vi "Drive Teleop Handler.vi"(10 "Call Context":T1) -> ()   [LabVIEW 2025]
uses:
  swerve-template/Type Definitions/Data/Robot Velocities.ctl
  <vilib>/Rock Robotics/WPI/DriverStation/WPI_DriverStationDerivedRobotMode.ctl
  Drive/Implementation/Driving Mode.ctl
  <vilib>/Rock Robotics/WPI/Joystick/XBox Buttons Indexer.ctl
  ce51abe2-3967-49ec-91df-d4b8ef358bb3.vi
  20f039dc-a6f5-4e97-88ba-31848a91c715.vi
  fdc21bd4-9215-41b8-8367-bf19dde4ba27.vi
  2558f998-dd4e-4154-8f44-6f70b21d0474.vi
  <vilib>/Rock Robotics/WPI/Utilities/WPI_GetSetVariantRefNum.vi
  <vilib>/Rock Robotics/Network Tables/NT Read Number.vi
  <vilib>/Rock Robotics/Network Tables/NT Read Boolean.vi
  Framework/Robot Global Data.vi
  <vilib>/Rock Robotics/Network Tables/NT Write Boolean.vi
panel:
  in  "Max Translation Align":dbl=4.0
  in  "Deadband Info":T2={"Deadband"=0.05, "Deadband High"=1.0, "Deadband Low"=0.05}
  in  "Max Velocities":T3={"X Velocity"=15.0, "Y Velocity"=15.0, "Rotational \nVelocity"=270.0}
  in  "Sinusoidal Terms":cluster{"Max Velocity":dbl, "Frequency":dbl}
  in  "Teleop Mode":T4(ring)
  in  "Joystick Inputs":T5(array[cluster])
  in  "Send Inputs":bool
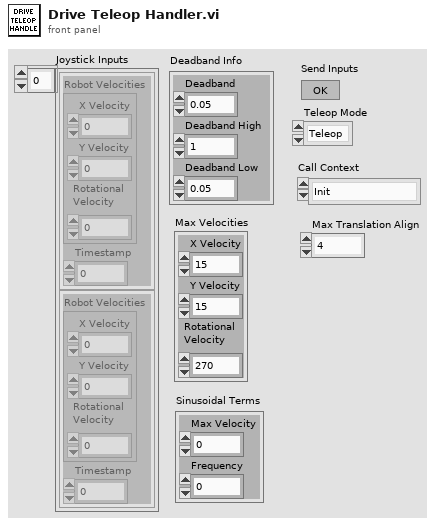
[diagram p1: front panel]
types:
  T1 = typedef "WPI_DriverStationDerivedRobotMode.ctl" = enum16{"Init", "Execute", "Stop"}
  T2 = cluster{"Deadband":dbl, "Deadband High":dbl, "Deadband Low":dbl}
  T3 = typedef "Robot Velocities.ctl" = cluster{"X Velocity":dbl, "Y Velocity":dbl, "Rotational \nVelocity":dbl}
  T4 = enum16{"Teleop", "Simulated Teleop", "Sine Velocity Profiles", "Circle Simulator"}
  T5 = cluster{"Robot Velocities":T3, "Timestamp":dbl}[]
  T6 = typedef "XBox Buttons Indexer.ctl" = enum16{"A", "B", "X", "Y", "Left Bumper", "Right Bumper", "Back", "Start", "Left Joystick", "Right Joystick"}
  T7 = typedef "Driving Mode.ctl" = enum16{"Robot Centric", "Field Centric"}
  T8 = typedef "WPI_JoystickDevRef.ctl" = cluster{"Device":T9}
  T9 = typedef "WPI_JoystickDeviceEnum.ctl" = enum16{"USB 0", "USB 1", "USB 2", "USB 3", "USB 4", "USB 5"}
  T10 = typedef "CTRE_PigeonIMU_DeviceRef.ctl" = cluster{"DeviceStatus":errorcluster, "Device Number":u8, "Type":T11, "Device ID":u32, "Handle":u64, "UsageFrame":u32, "Library Path":path}
  T11 = typedef "CTRE_PigeonIMU_ConnectionType.ctl" = u32
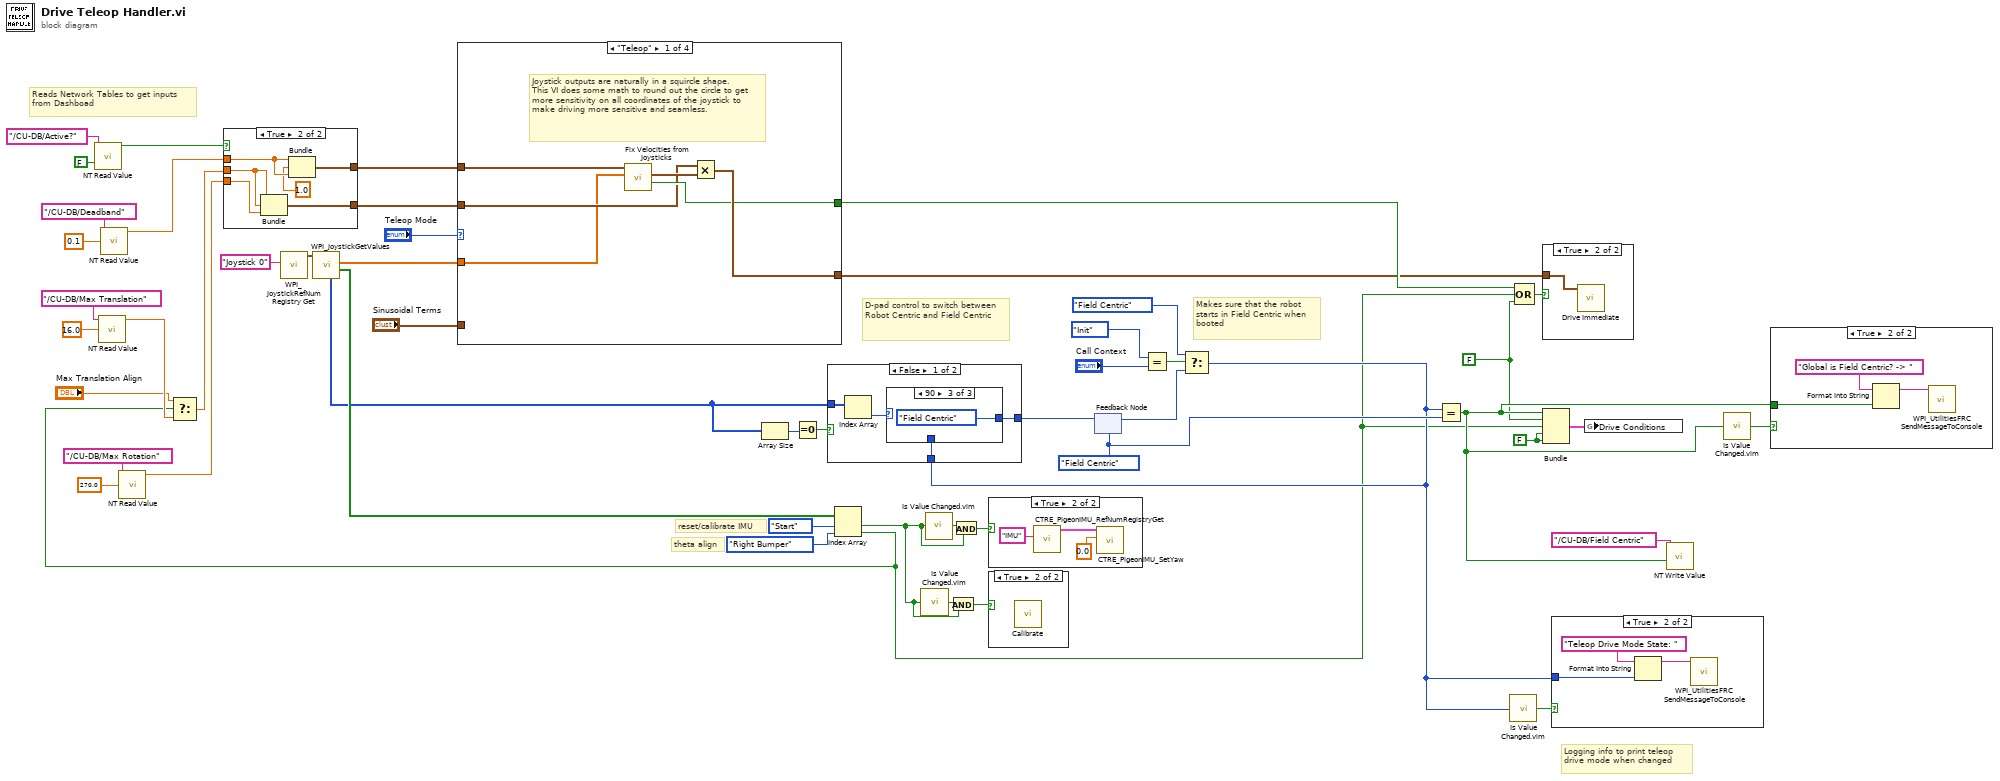
[diagram p0: block diagram]
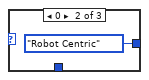
[diagram p7: hidden frame]
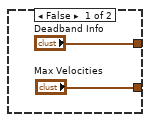
[diagram p9: hidden frame]
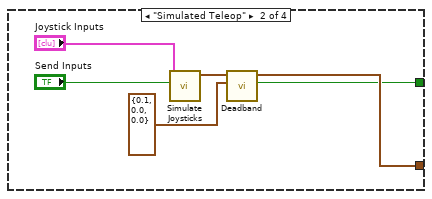
[diagram p10: hidden frame]
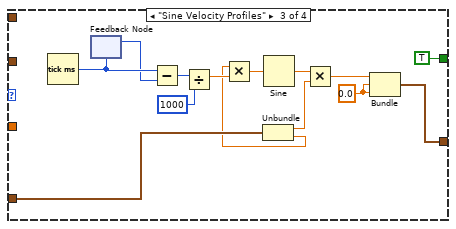
[diagram p11: hidden frame]
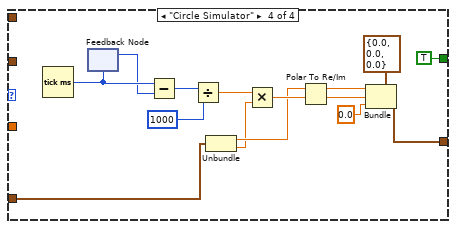
[diagram p12: hidden frame]
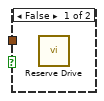
[diagram p13: hidden frame]
diagram:
  w6 = FALSE
  w5 = FALSE
  w18 = Driving_Mode."Field Centric"
  # "theta align"
  # "reset/calibrate IMU"
  # "Reads Network Tables to get inputs from Dashboad"
  # "Logging info to print teleop drive mode when changed"
  # "Makes sure that the robot starts in Field Centric when booted"
  # "D-pad control to switch between Robot Centric and Field Centric"
  n1 = call-poly <vilib>:"NT Read Value.vi"("default value"=FALSE ("Default Value"), "name"="/CU-DB/Active?" ("Name")) -> ("value"=w33:bool)  [unwired: 7 in, 2 out]
  n2 = call-poly <vilib>:"NT Read Value.vi"("default value"=16.0 ("Default Value"), "name"="/CU-DB/Max Translation" ("Name")) -> ("value"=w3:dbl)  [unwired: 7 in, 2 out]
  n3 = call-poly <vilib>:"NT Read Value.vi"("default value"=0.1 ("Default Value"), "name"="/CU-DB/Deadband" ("Name")) -> ("value"=w32:dbl)  [unwired: 7 in, 2 out]
  n4 = call-poly <vilib>:"NT Read Value.vi"("default value"=270.0 ("Default Value"), "name"="/CU-DB/Max Rotation" ("Name")) -> ("value"=w30:dbl)  [unwired: 7 in, 2 out]
  n5 = call <vilib>:"WPI_JoystickRefNum Registry Get.vi"("refnum name"="Joystick 0") -> ("JoystickDevRef"=w50:T8)  [unwired: 1 in, 9 out]
  n6 = call <vilib>:"WPI_JoystickGetValues.vi"("JoystickDevRef"=w50) -> ("Buttons"=w47:bool[], "Axes"=w49:dbl[], "POVs"=w25:i16[])  [unwired: 6 in, 2 out]
  n7 = Array Size(array=w25) -> (size(s)=w24:i32)
  n8 = Equal To 0?(x=w24) -> (x = 0?=w23:bool)
  n9 = Index Array(array=w47, index #1=XBox_Buttons_Indexer."Start" ("XBox Buttons"), index #2=XBox_Buttons_Indexer."Right Bumper" ("XBox Buttons")) -> (element #1=w10:bool, element #2=w2:bool)
  n10 = Select(t="Max Translation Align", s=w2, f=w3) -> (s? t:f=w4:dbl)
  n11 = case shown="True" w33 {
    tunnel: w32 -> [_ w59]
    tunnel: ["Deadband Info" w57] -> w31
    tunnel: w4 -> [_ w56]
    tunnel: w30 -> [_ w55]
    tunnel: ["Max Velocities" w54] -> w29
    frame False {
    }
    frame True {
      n12 = Bundle("value"=w56, "value"=w56, "value"=w55) -> (w54:cluster{"value":dbl, "value":dbl, "value":dbl})  [unwired: 1 in]
      n13 = Bundle("value"=w59, "value"=1.0, "value"=w59) -> (w57:cluster{"value":dbl, "value":dbl, "value":dbl})  [unwired: 1 in]
    }
  }
  n14 = case shown="\"Teleop\"" "Teleop Mode" {
    tunnel: w49 -> [w60 _ _ _]
    tunnel: [w65 w71 w76 w98] -> w8
    tunnel: "Sinusoidal Terms" -> [_ _ w75 w88]
    tunnel: w31 -> [w64 _ _ _]
    tunnel: w29 -> [w61 _ _ _]
    tunnel: [w62 w66 TRUE ("Sending Input?") TRUE ("Sending Input?")] -> w27
    frame "Teleop" {
      # "Joystick outputs are naturally in a squircle shape.\nThis VI does some math to round out the circle to get more sensitivity on all coordinates of the joystick to make driving more sensitive and seamless."
      n15 = call "Fix Velocities from Joysticks.vi"("Axes"=w60, "Deadband"=w64) -> ("Sending Input?"=w62:bool, "Adjusted Robot Velocities"=w63:T3)  [unwired: 8 in]
      n16 = Multiply(x=w61, y=w63) -> (x*y=w65:T3)
    }
    frame "Simulated Teleop" {
      n17 = call "Simulate Joysticks.vi"("Send Inputs"="Send Inputs", "Joystick Inputs"="Joystick Inputs") -> ("Joystick Inputs"=w68:T3)  [unwired: 9 in]
      n18 = call "Deadband.vi"("Deadband Info"=T2 {"Deadband"=0.1, "Deadband High"=0.0, "Deadband Low"=0.0}, "Robot Velocities"=w68) -> ("Sending Input?"=w66:bool, "Adjusted Robot Velocities"=w71:T3)  [unwired: 8 in]
    }
    frame "Sine Velocity Profiles" {
      w84 = 0.0
      n19 = Tick Count (ms)() -> (millisecond timer value=w78:u32)
      n20 = feedback #1(w78) -> (w77:u32)
      n21 = feedback-in #1(w77) -> ()
      n22 = Subtract(x=w78, y=w77) -> (x-y=w82:u32)
      n23 = Divide(x=w82, y=u32 1000) -> (x/y=w80:dbl)
      n24 = Unbundle(w75) -> ("Max Velocity"=w73:dbl, "Frequency"=w74:dbl)
      n25 = Multiply(x=w74, y=w80) -> (x*y=w79:dbl)
      n26 = Sine(x=w79) -> (sin(x)=w83:dbl)
      n27 = Multiply(x=w83, y=w73) -> (x*y=w85:dbl)
      n28 = Bundle(w85, w84, w84) -> (w76:cluster{dbl, dbl, dbl})  [unwired: 1 in]
    }
    frame "Circle Simulator" {
      n29 = Tick Count (ms)() -> (millisecond timer value=w94:u32)
      n30 = feedback #2(w94) -> (w93:u32)
      n31 = feedback-in #2(w93) -> ()
      n32 = Subtract(x=w94, y=w93) -> (x-y=w96:u32)
      n33 = Divide(x=w96, y=u32 1000) -> (x/y=w90:dbl)
      n34 = Unbundle(w88) -> ("Max Velocity"=w91:dbl, "Frequency"=w89:dbl)
      n35 = Multiply(x=w90, y=w89) -> (x*y=w92:dbl)
      n36 = Polar To Re/Im(2:w92, 3:w91) -> (0:w86:dbl, 1:w87:dbl)
      n37 = Bundle(cluster=T3 {"X Velocity"=0.0, "Y Velocity"=0.0, "Rotational \nVelocity"=0.0} ("Robot Velocities (ft/s and deg/s)"), "X Velocity"=w87, "Y Velocity"=w86, "Rotational \nVelocity"=0.0 ("Rotational \nVelocity")) -> (w98:T3)
    }
  }
  n38 = call "Is Value Changed.vim"("value"=w10) -> ("changed or first call?"=w13:bool)
  n39 = call "Is Value Changed.vim"("value"=w10) -> ("changed or first call?"=w45:bool)
  n40 = And(x=w13, y=w10) -> (x .and. y?=w12:bool)
  n41 = And(x=w45, y=w10) -> (x .and. y?=w44:bool)
  n42 = case shown="True" w44 {
    frame False {
    }
    frame True {
      n43 = call <vilib>:"CTRE_PigeonIMU_RefNumRegistryGet.vi"("refnum name"="IMU") -> ("PigeonIMUDevRef"=w102:T10)  [unwired: 9 in, 1 out]
      n44 = call <vilib>:"CTRE_PigeonIMU_SetYaw.vi"("Value"=0.0, "PigeonIMUDevRef"=w102) -> ()  [unwired: 8 in, 2 out]
    }
  }
  n45 = case shown="True" w12 {
    frame False {
    }
    frame True {
      n46 = call "Calibrate.vi"() -> ()  [unwired: 11 in, 1 out]
    }
  }
  n47 = feedback #3(w18) -> (w17:T7)
  n48 = Equal?(x=WPI_DriverStationDerivedRobotMode."Init" ("y"), y="Call Context") -> (x = y?=w20:bool)
  n49 = Select(t=Driving_Mode."Field Centric" ("x"), s=w20, f=w17) -> (s? t:f=w15:T7)
  n50 = case shown="False" w23 {
    tunnel: [w106 w111] -> w48
    tunnel: w15 -> [w105 w111]
    tunnel: w25 -> [w104 _]
    frame False {
      n51 = Index Array(array=w104) -> (element=w107:i16)  [unwired: 1 in]
      n52 = case shown="90" w107 {
        tunnel: [w108 Driving_Mode."Robot Centric" Driving_Mode."Field Centric"] -> w106
        tunnel: w105 -> [w108 _ _]
        frame -1, Default {
        }
        frame 0 {
        }
        frame 90 {
        }
      }
    }
    frame True {
    }
  }
  n53 = feedback-in #3(w48) -> ()
  n54 = Equal?(x=w15, y=w18) -> (x = y?=w7:bool)
  n55 = call "Is Value Changed.vim"("value"=w15) -> ("changed or first call?"=w14:bool)
  n56 = Compound Arithmetic op=OR(w27, w2, w6) -> (w28:bool)
  n57 = case shown="True" w28 {
    tunnel: w8 -> [_ w112]
    frame False {
      n58 = call "Reserve Drive.vi"() -> ()  [unwired: 11 in, 1 out]
    }
    frame True {
      n59 = call "Drive Immediate.vi"("Robot Velocities"=w112) -> ()  [unwired: 10 in, 1 out]
    }
  }
  n60 = Bundle(w7, w6, w2, w5, w5) -> (w11:cluster{bool, bool, bool, bool, bool})  [unwired: 1 in]
  n61 = case shown="True" w14 {
    tunnel: w15 -> [_ w113]
    frame False {
    }
    frame True {
      n62 = Format Into String(initial string="Teleop Drive Mode State: ", w113) -> (resulting string=w115:string)  [unwired: 2 in, 1 out]
      n63 = call <vilib>:"WPI_UtilitiesFRC SendMessageToConsole.vi"("Message"=w115) -> ()  [unwired: 14 in, 1 out]
    }
  }
  n64 = global write "Robot Global Data.vi" "Drive Conditions"(w11) -> ()
  n65 = call-poly <vilib>:"NT Write Value.vi"("value"=w7, "name"="/CU-DB/Field Centric") -> ()  [unwired: 9 in, 1 out]
  n66 = call "Is Value Changed.vim"("value"=w7) -> ("changed or first call?"=w16:bool)
  n67 = case shown="True" w16 {
    tunnel: w7 -> [_ w117]
    frame False {
    }
    frame True {
      n68 = Format Into String(initial string="Global is Field Centric? -> ", w117) -> (resulting string=w118:string)  [unwired: 2 in, 1 out]
      n69 = call <vilib>:"WPI_UtilitiesFRC SendMessageToConsole.vi"("Message"=w118) -> ()  [unwired: 14 in, 1 out]
    }
  }
